vi "Decoration - Workspace Color Control.vi"() -> ()   [LabVIEW 2013]
doc: "Sample numeric display item."
uses:
  <vilib>/NI Veristand/Display Template Support/Display Template Support.llb/cluster_Screen Item Settings.ctl
  <vilib>/NI Veristand/Display Template Support/Display Template Support.llb/cluster_Graph Scale Settings.ctl
  <vilib>/NI Veristand/Display Template Support/Display Template Support.llb/cluster_Graph Plot Settings.ctl
  <vilib>/NI Veristand/Display Template Support/Display Template Support.llb/enum_Display Template Handler Minimal To Widget Msg.ctl
  <vilib>/NI Veristand/Display Template Support/Display Template Support.llb/enum_Display Template Handler Minimal To Workspace.ctl
panel:
  in  "Workspace Color":u32(colorbox)
  in  "Item.Data":T1
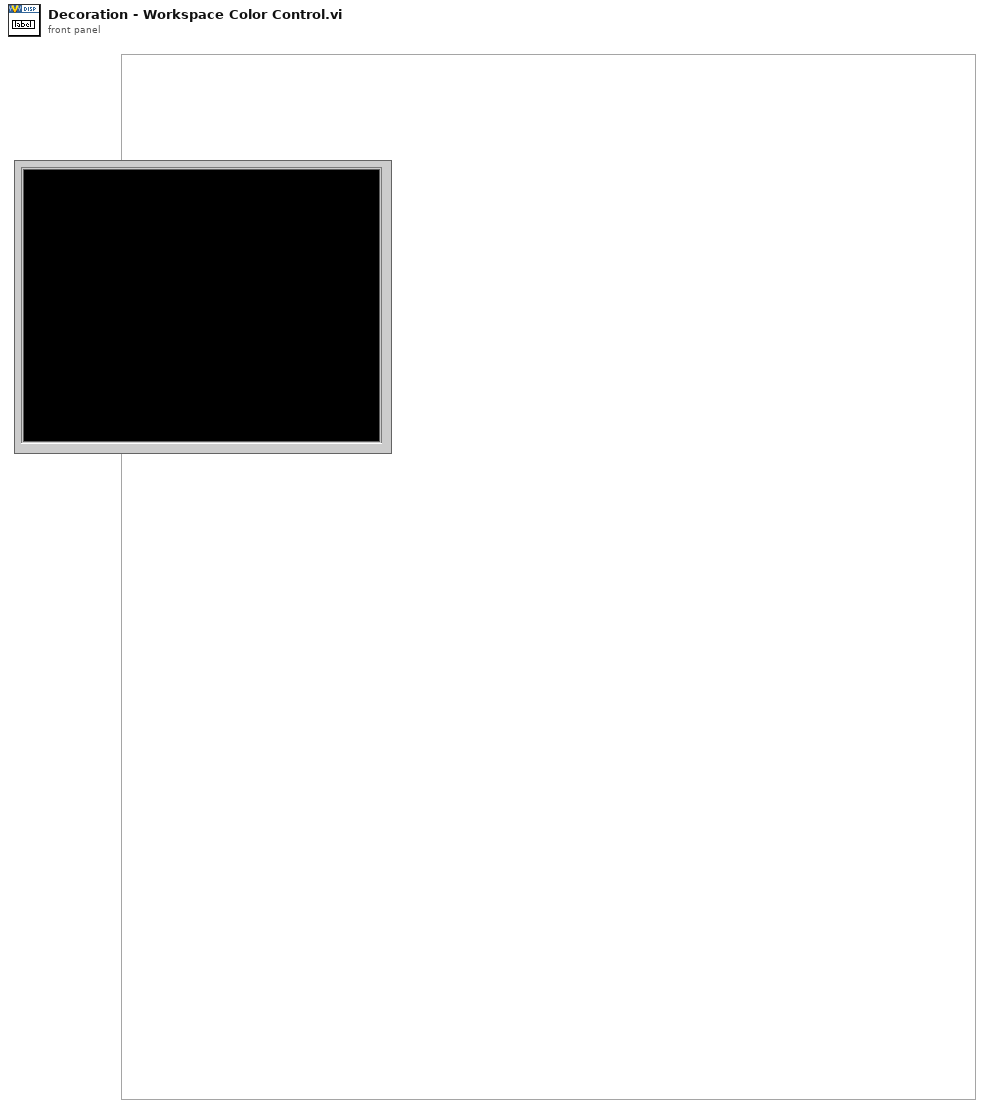
[diagram p1: front panel]
types:
  T1 = typedef "cluster_Screen Item Settings.ctl" = cluster{"Template VI":string, "Position X":i32, "Position Y":i32, "Custom":string, "Show Title Bar":bool, "ID":i32, "Always On Top":bool, "Allow Resize":bool, "Allow Minimize":bool, "Allow Close":bool, "Size to Screen":bool, "Screen.ID":i32, "State":enum16{"Normal", "New"}, "Title":string, "Window Bounds":cluster{"[0]":i16, "[1]":i16, "[2]":i16, "[3]":i16}, "Channel Ref":u64, "Unit":string, "Default Units?":bool, "Flash Limit?":bool, "Color 1":u32, "Color 2":u32, "Color 3":u32, "Color 4":u32, "Bck Color":u32, "Fore Color":u32, "Limit 1":dbl, "Limit 2":dbl, "Limit 3":dbl, "Limit 4":dbl, "Limit Mode 1":i32, "Limit Mode 2":i32, "Limit Mode 3":i32, "Limit Mode 4":i32, "Scale Precision":i32, "Scale Min":dbl, "Scale Max":dbl, "Format":i32, "Precision":i32, "Background Type":i32, "IDs":i32[], "Units":string[], "Labels":string[], "Scale Factor":dbl, "Scale Offset":dbl, "YScale Index":u32[], "XScale":T2, "YScales":T2[], "Plots":T3[], "Update Period":dbl, "History Length":dbl, "My.Ref":refnum<vi>, "Is Control?":bool, "Channel Paths":string[], "Custom Data":variant}
  T2 = typedef "cluster_Graph Scale Settings.ctl" = cluster{"Format":u8, "Precision":u8, "Fit":u8, "Label":string, "Use Default Label":bool, "Label Visible":bool, "Min":dbl, "Max":dbl}
  T3 = typedef "cluster_Graph Plot Settings.ctl" = cluster{"Bar Style":u8, "Fill To":i16, "Fill/PtColor":u32, "Line Style":u8, "Line Width":u8, "Color":u32, "Interp":u8, "Point Style":u8}
  T4 = typedef "enum_Display Template Handler Minimal To Workspace.ctl" = cluster{"Operation":enum16{"SetCustomData", "DeleteItem"}, "Data":variant}
  T5 = typedef "enum_Display Template Handler Minimal To Widget Msg.ctl" = enum16{"Stop", "LaunchConfigDialog"}
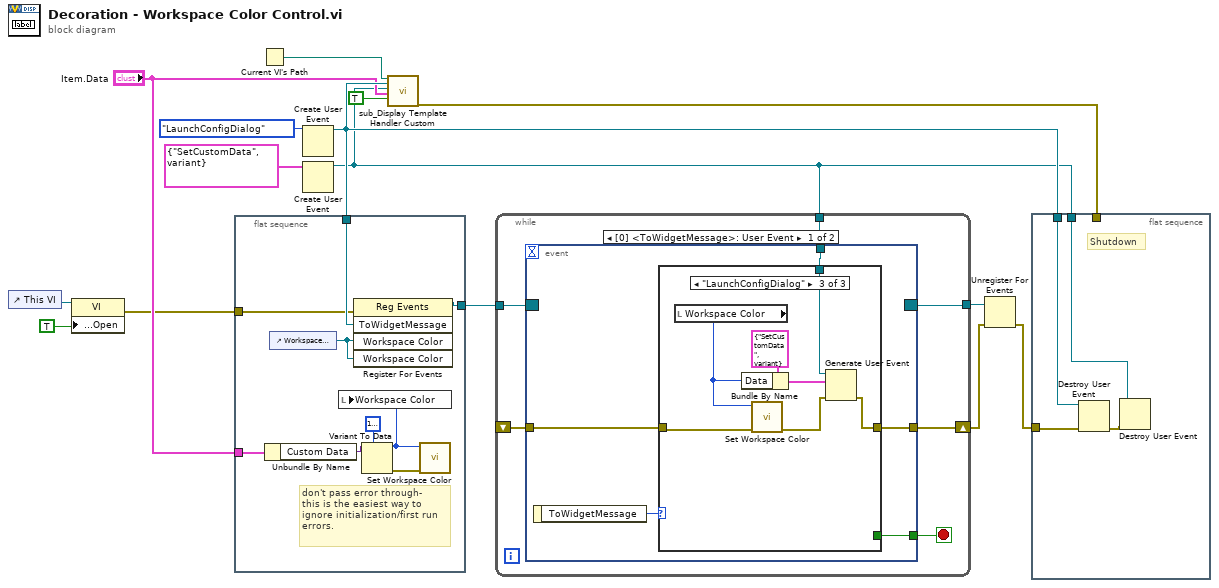
[diagram p0: block diagram]
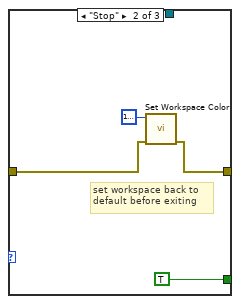
[diagram p3: hidden frame]
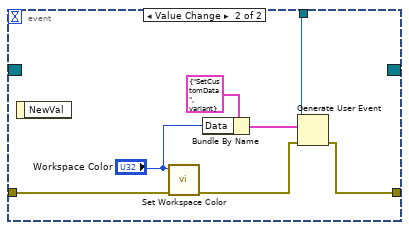
[diagram p4: hidden frame]
diagram:
  n1 = control-ref of="This VI"() -> (w4:refnum<vi>)
  n2 = property class="VI"(reference=w4, "Front Panel.Open"=TRUE ("Front Panel Window:Open")) -> (error out=w2:errorcluster)  [unwired: 1 in, 1 out]
  n3 = flat-sequence {
    tunnel: [w19] -> w13
    tunnel: w10 -> [w18]
    tunnel: "Item.Data" -> [w24]
    tunnel: w2 -> [w16]
    frame #0 {
      # "don't pass error through-\nthis is the easiest way to\nignore initialization/first run\nerrors."
      n4 = Unbundle By Name(w24) -> ("Custom Data"=w23:variant)
      n5 = control-ref of="Workspace Color"() -> (w17:refnum<vi>)
      n6 = register-events(error in=w16, w18, w17, w17) -> (reference out=w19:refnum<event-registration>)  [unwired: 1 in, 1 out]
      n7 = Variant To Data(type=u32 16777225, Variant=w23) -> (data=w20:u32, error out=w21:errorcluster)  [unwired: 1 in]
      n8 = local write "Workspace Color"(w20) -> ()
      n9 = call "Set Workspace Color.vi"("Error In"=w21, "Color to set"=w20) -> ()  [unwired: 9 in, 1 out]
    }
  }
  n10 = Current VI's Path() -> (path=w8:path)
  n11 = Create User Event(user event datatype=enum_Display_Template_Handler_Minimal_To_Widget_Msg."LaunchConfigDialog" ("ToWidgetMessage")) -> (user event=w10:refnum<user-event>)  [unwired: 1 in, 1 out]
  n12 = Create User Event(user event datatype=T4 {"Operation"=enum."SetCustomData", "Data"=variant} ("Data")) -> (user event=w5:refnum<user-event>)  [unwired: 1 in, 1 out]
  n13 = call <vilib>:"sub_Display Template Handler Custom.vi"("Parent.Path"=w8, "ToWidgetEvent"=w10, "ToWorkspace"=w5, "Item.Data"="Item.Data", "Resizable"=TRUE) -> ("error out"=w15:errorcluster)  [unwired: 14 in]
  n14 = while {
    tunnel: w13 -> [w30]
    tunnel: [w28] -> w12
    shift-right: [w27] -> w1
    shift-left: _ -> [w25]
    tunnel: w5 -> [w26]
    stop <- w29 stop-if-true
    n15 = event shown="[0] <ToWidgetMessage>: User Event" {
      selector: w30 -> [_ _]
      dyn-events: [_ _] -> w28
      timeout: _ -> [_ _]
      tunnel: [w34 _] -> w29
      tunnel: w25 -> [w31 w54]
      tunnel: [w33 w50] -> w27
      tunnel: w26 -> [w32 w48]
      event User Event {
        n16 = event-data() -> ("ToWidgetMessage"=w35:T5)  [unwired: 1 out]
        n17 = case shown="\"LaunchConfigDialog\"" w35 {
          tunnel: [_ TRUE _] -> w34
          tunnel: [w36 w39 w41] -> w33
          tunnel: w31 -> [w36 w37 w45]
          tunnel: w32 -> [_ _ w42]
          frame Default {
          }
          frame "Stop" {
            # "set workspace back to \ndefault before exiting"
            n18 = call "Set Workspace Color.vi"("Error In"=w37, "Color to set"=u32 16777226) -> ("Error Out"=w39:errorcluster)  [unwired: 9 in]
          }
          frame "LaunchConfigDialog" {
            n19 = local read "Workspace Color"() -> (w43:u32)
            n20 = Bundle By Name(cluster=T4 {"Operation"=enum."SetCustomData", "Data"=variant} ("event data"), "Data"=w43) -> (w46:T4)
            n21 = call "Set Workspace Color.vi"("Error In"=w45, "Color to set"=w43) -> ("Error Out"=w44:errorcluster)  [unwired: 9 in]
            n22 = Generate User Event(user event=w42, event data cluster=w46, error in=w44) -> (error out=w41:errorcluster)  [unwired: 1 in, 1 out]
          }
        }
      }
      event Value Change {
        n23 = event-data() -> ()  [unwired: 2 out]
        n24 = call "Set Workspace Color.vi"("Error In"=w54, "Color to set"="Workspace Color") -> ("Error Out"=w51:errorcluster)  [unwired: 9 in]
        n25 = Bundle By Name(cluster=T4 {"Operation"=enum."SetCustomData", "Data"=variant} ("event data"), "Data"="Workspace Color") -> (w52:T4)
        n26 = Generate User Event(user event=w48, event data cluster=w52, error in=w51) -> (error out=w50:errorcluster)  [unwired: 1 in, 1 out]
      }
    }
  }
  n27 = Unregister For Events(event registration refnum=w12, error in=w1) -> (error out=w11:errorcluster)
  n28 = flat-sequence {
    tunnel: w15 -> [_]
    tunnel: w11 -> [w57]
    tunnel: w10 -> [w58]
    tunnel: w5 -> [w55]
    frame #0 {
      # "Shutdown"
      n29 = Destroy User Event(user event=w58, error in=w57) -> (error out=w56:errorcluster)
      n30 = Destroy User Event(user event=w55, error in=w56) -> ()  [unwired: 1 out]
    }
  }
